vi "test_libssh2_session_methods.vi"() -> ()   [LabVIEW 2017, in "integration_tests.lvlib"]
uses:
  integration_tests.lvlib
  libssh2/libssh2_method_type.ctl
  libssh2/libssh2_session_handshake_tcp.vi
  libssh2/libssh2_init_default.vi
  libssh2/libssh2_session_init_ex.vi
  <vilib>/Utility/tcp.llb/TCP Get Raw Net Object.vi
  libssh2/libssh2_session_handshake_socket.vi
  libssh2/libssh2.lvlib
  support/support.lvlib
  <vilib>/PNR/Transparent Assertions/Transparent Assertions/Transparent Assertions.lvlib
panel:
  out "error out":errorcluster
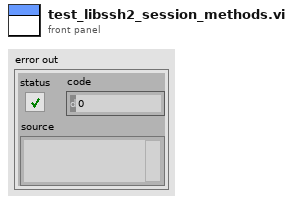
[diagram p1: front panel]
types:
  T1 = typedef "libssh2.lvlib/libssh2_method_type.ctl" = enum16{"LIBSSH2_METHOD_KEX", "LIBSSH2_METHOD_HOSTKEY", "LIBSSH2_METHOD_CRYPT_CS", "LIBSSH2_METHOD_CRYPT_SC", "LIBSSH2_METHOD_MAC_CS", "LIBSSH2_METHOD_MAC_SC", "LIBSSH2_METHOD_COMP_CS", "LIBSSH2_METHOD_COMP_SC", "LIBSSH2_METHOD_LANG_CS", "LIBSSH2_METHOD_LANG_SC", "LIBSSH2_METHOD_SIGN_ALGO"}
  T2 = typedef "libssh2.lvlib/Session Refnum.ctl" = refnum<k1>
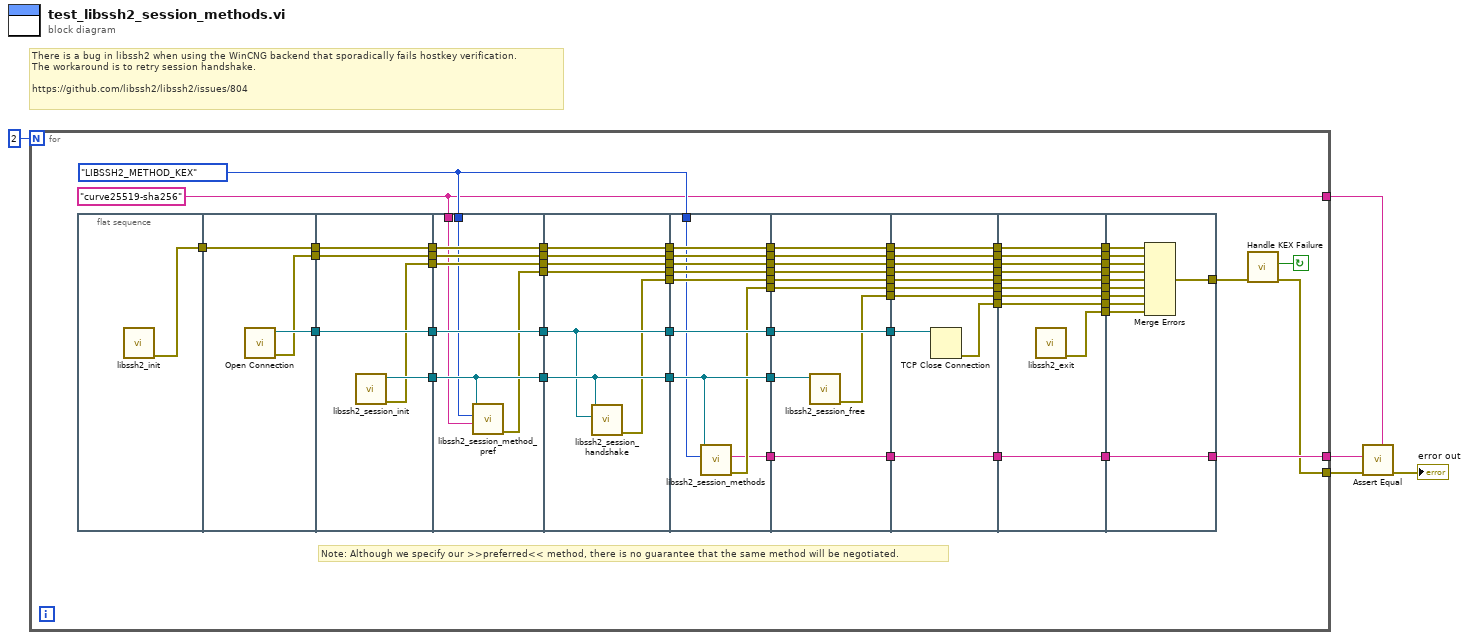
[diagram p0: block diagram]
diagram:
  # "There is a bug in libssh2 when using the WinCNG backend that sporadically fails hostkey verification.\nThe workaround is to retry session handshake.\n\nhttps://github.com/libssh2/libssh2/issues/804"
  n1 = for {
    N: 2 -> [_]
    tunnel: [w7] -> w5
    tunnel: [w10] -> w3
    tunnel: [w9] -> w2
    stop <- w6 continue-if-true
    w11 = libssh2_method_type."LIBSSH2_METHOD_KEX" ("method_type")
    w10 = "curve25519-sha256"
    # "Note: Although we specify our >>preferred<< method, there is no guarantee that the same method will be negotiated."
    n2 = flat-sequence {
      tunnel: [w71] -> w70
      tunnel: [w74] -> w69
      tunnel: w70 -> [w73]
      tunnel: [w73] -> w68
      tunnel: [w72] -> w67
      tunnel: w69 -> [w79]
      tunnel: [w79] -> w66
      tunnel: w68 -> [w78]
      tunnel: [w78] -> w65
      tunnel: w67 -> [w77]
      tunnel: [w77] -> w64
      tunnel: [w76] -> w63
      tunnel: [w75] -> w62
      tunnel: w66 -> [w87]
      tunnel: [w87] -> w61
      tunnel: w65 -> [w86]
      tunnel: [w86] -> w60
      tunnel: w64 -> [w85]
      tunnel: [w85] -> w59
      tunnel: w63 -> [w83]
      tunnel: [w83] -> w58
      tunnel: w62 -> [w84]
      tunnel: [w84] -> w57
      tunnel: [w82] -> w56
      tunnel: w11 -> [w81]
      tunnel: w10 -> [w80]
      tunnel: w61 -> [w90]
      tunnel: [w90] -> w55
      tunnel: w60 -> [w94]
      tunnel: [w94] -> w54
      tunnel: w59 -> [w93]
      tunnel: [w93] -> w53
      tunnel: [w92] -> w52
      tunnel: w58 -> [w92]
      tunnel: w57 -> [w91]
      tunnel: [w91] -> w51
      tunnel: [w89] -> w50
      tunnel: w56 -> [w88]
      tunnel: [w88] -> w49
      tunnel: w55 -> [w104]
      tunnel: [w104] -> w48
      tunnel: w54 -> [w103]
      tunnel: [w103] -> w47
      tunnel: w53 -> [w102]
      tunnel: [w102] -> w46
      tunnel: w52 -> [w98]
      tunnel: [w98] -> w45
      tunnel: w51 -> [w101]
      tunnel: [w101] -> w44
      tunnel: [w96] -> w43
      tunnel: w50 -> [w100]
      tunnel: [w100] -> w42
      tunnel: [w97] -> w41
      tunnel: w49 -> [w99]
      tunnel: [w99] -> w40
      tunnel: w11 -> [w95]
      tunnel: w48 -> [w114]
      tunnel: [w114] -> w39
      tunnel: w47 -> [w113]
      tunnel: [w113] -> w38
      tunnel: w46 -> [w112]
      tunnel: [w112] -> w37
      tunnel: w45 -> [w111]
      tunnel: w44 -> [w110]
      tunnel: [w110] -> w36
      tunnel: [w109] -> w35
      tunnel: w43 -> [w108]
      tunnel: [w108] -> w34
      tunnel: w42 -> [w107]
      tunnel: [w107] -> w33
      tunnel: w41 -> [w106]
      tunnel: [w106] -> w32
      tunnel: w40 -> [w105]
      tunnel: [w105] -> w31
      tunnel: w39 -> [w124]
      tunnel: w38 -> [w123]
      tunnel: [w123] -> w30
      tunnel: w37 -> [w122]
      tunnel: [w122] -> w29
      tunnel: [w121] -> w28
      tunnel: w36 -> [w120]
      tunnel: [w120] -> w27
      tunnel: w35 -> [w119]
      tunnel: [w119] -> w26
      tunnel: w34 -> [w118]
      tunnel: [w118] -> w25
      tunnel: w33 -> [w117]
      tunnel: [w117] -> w24
      tunnel: w32 -> [w116]
      tunnel: [w116] -> w23
      tunnel: w31 -> [w115]
      tunnel: [w115] -> w22
      tunnel: w30 -> [w134]
      tunnel: [w134] -> w21
      tunnel: w29 -> [w133]
      tunnel: [w133] -> w20
      tunnel: w28 -> [w132]
      tunnel: [w132] -> w19
      tunnel: [w131] -> w18
      tunnel: w27 -> [w130]
      tunnel: [w130] -> w17
      tunnel: w26 -> [w129]
      tunnel: [w129] -> w16
      tunnel: w25 -> [w128]
      tunnel: [w128] -> w15
      tunnel: w24 -> [w127]
      tunnel: [w127] -> w14
      tunnel: w23 -> [w126]
      tunnel: [w126] -> w13
      tunnel: w22 -> [w125]
      tunnel: [w125] -> w12
      tunnel: w21 -> [w145]
      tunnel: w20 -> [w144]
      tunnel: w19 -> [w143]
      tunnel: w18 -> [w142]
      tunnel: w17 -> [w141]
      tunnel: w16 -> [w140]
      tunnel: w15 -> [w136]
      tunnel: [w135] -> w8
      tunnel: w14 -> [w139]
      tunnel: w13 -> [w138]
      tunnel: w12 -> [w137]
      tunnel: [w136] -> w9
      frame #0 {
        n3 = call-poly "libssh2_init.vi"() -> ("error out"=w71:errorcluster)  [unwired: 11 in]
      }
      frame #1 {
        n4 = call "Open Connection.vi"() -> ("error out"=w72:errorcluster, "connection ID"=w74:refnum<k5>)  [unwired: 10 in]
      }
      frame #2 {
        n5 = call "libssh2_session_init.vi"() -> ("error out"=w75:errorcluster, "session"=w76:T2)  [unwired: 10 in]
      }
      frame #3 {
        n6 = call "libssh2_session_method_pref.vi"("prefs"=w80, "method_type"=w81, "session"=w83) -> ("error out"=w82:errorcluster)  [unwired: 8 in]
      }
      frame #4 {
        n7 = call-poly "libssh2_session_handshake.vi"("tcp connection"=w90, "session"=w92) -> ("error out"=w89:errorcluster)  [unwired: 9 in]
      }
      frame #5 {
        n8 = call "libssh2_session_methods.vi"("method_type"=w95, "session"=w98) -> ("error out"=w97:errorcluster, "methods"=w96:string)  [unwired: 8 in]
      }
      frame #6 {
        n9 = call "libssh2_session_free.vi"("session"=w111) -> ("error out"=w109:errorcluster)  [unwired: 10 in]
      }
      frame #7 {
        n10 = TCP Close Connection(connection ID=w124) -> (error out=w121:errorcluster)  [unwired: 2 in, 1 out]
      }
      frame #8 {
        n11 = call "libssh2_exit.vi"() -> ("error out"=w131:errorcluster)  [unwired: 11 in]
      }
      frame #9 {
        n12 = Merge Errors(w145, w144, w141, w137, w139, w138, w140, w143, w142) -> (w135:errorcluster)
      }
    }
    n13 = call "Handle KEX Failure.vi"("error in (no error)"=w8) -> ("error out"=w7:errorcluster, "KEX Failure"=w6:bool)  [unwired: 9 in]
  }
  n14 = call <vilib>:"Assert Equal.vi"("Expected"=w3, "error in (no error)"=w5, "Actual"=w2) -> ("error out"=→"error out":errorcluster)  [unwired: 8 in]
